vi "Close.vi"(8 "error in (no error)":errorcluster, 11 "hdl":i32) -> (0 "error out":errorcluster)   [LabVIEW 2013, in "Thorlabs_MC2000B.lvlib"]
uses:
  <instrlib>/Thorlabs_MC2000B/Thorlabs_MC2000B.lvlib
  <instrlib>/Thorlabs_MC2000B/Library/MC2000CommandLibWin64.dll
  <instrlib>/Thorlabs_MC2000B/Library/MC2000CommandLibWin32.dll
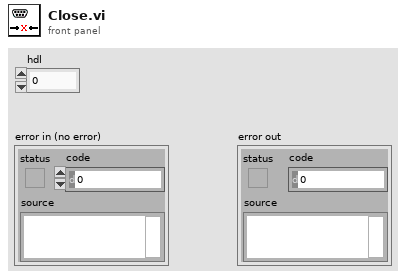
[diagram p1: front panel]
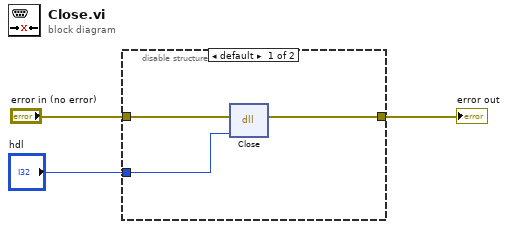
[diagram p0: block diagram]
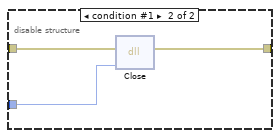
[diagram p2: hidden frame]
diagram:
  n1 = disable-structure shown="default" {
    disable-tunnel: "error in (no error)" -> [w6 w9]
    disable-tunnel: [w5 w8] -> w2
    disable-tunnel: "hdl" -> [w4 w7]
    frame condition #0 (active) {
      n2 = dll-call lib="C:/Program Files (x86)/National Instruments/LabVIEW 2013/instr.lib/Thorlabs_MC2000B/Library/MC2000CommandLibWin32.dll" fn="Close"(error in=w6, "hdl"=w4) -> (error out=w5:errorcluster)  [unwired: 4 in, 1 out]
    }
    frame condition #1 {
      n3 = dll-call lib="D:/Program Files/National Instruments/LabVIEW 2011/instr.lib/Thorlabs_MC2000B/Library/MC2000CommandLibWin64.dll" fn="Close"(error in=w9, "hdl"=w7) -> (error out=w8:errorcluster)  [unwired: 4 in, 1 out]
    }
  }
  "error out" <- w2
